vi "CPU Average.vi"(8 "error in (no error)":errorcluster, 9 "error IO":errorcluster, 10 "CPU1 use":dbl, 11 "CPU0 use":dbl) -> (0 "error out":errorcluster, 3 "Average CPU use":dbl)   [LabVIEW 2016, in "Top Level.lvlib"]
uses:
  Top Level.lvlib
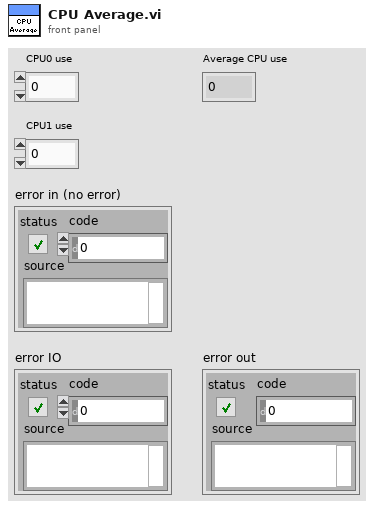
[diagram p1: front panel]
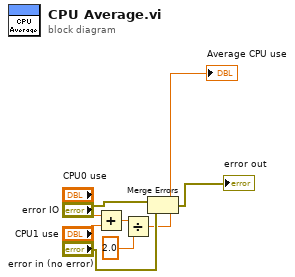
[diagram p0: block diagram]
diagram:
  n1 = Add(x="CPU0 use", y="CPU1 use") -> (x+y=w3:dbl)
  n2 = Divide(x=w3, y=2.0) -> (x/y=→"Average CPU use":dbl)
  n3 = Merge Errors("error IO", "error in (no error)") -> (→"error out":errorcluster)
